vi "BassybassMode.vi"(8 "error in":errorcluster) -> ()   [LabVIEW 2018]
doc: "This VI runs in parallel to other tasks. It can contain as many user-defined periodic loops as you need. These can carry out PID or other sorts of timed response."
uses:
  <vilib>/Platform/TimedLoop/XDataNode/timing_clust.ctl
  <vilib>/Platform/TimedLoop/XDataNode/nitl_modes.ctl
  <vilib>/Platform/TimedLoop/XDataNode/wakeup.ctl
  <vilib>/addons/control/pid/pid.llb/PID (DBL).vi
  <vilib>/platform/TimedLoop/XDataNode/XDataNode.xnode
  <vilib>/addons/control/pid/NI_PID_pid.lvlib
  <vilib>/Platform/TimedLoop/XDataNode/XDNodeRunTimeDep.lvlib
  <vilib>/Rock Robotics/Network Tables/NT Read Numeric Array.vi
panel:
  out "Distance (in)":dbl(slide) scale=14.0..50.0
  in  "XY Tail":i32=10
  out "XY Graph":cluster{dbl[], dbl[]}(graph)
  in  "Moving Avg Size":i32=4
  out "X":cluster{"Numeric":dbl, dbl}(graph)
  out "Z":cluster{"Numeric":dbl, dbl}(graph)
  out "Avg Z":dbl
  out "Avg X":dbl
  out "Cam Tran Array":dbl[](array[numeric])
  out "Yaw Wrap":dbl(graph)=90.04595407731806
  out "Cal Status":T1={"Mag"={"[0]"=FALSE, "[1]"=FALSE, "[2]"=FALSE, "[3]"=TRUE}, "Acc"={"[0]"=TRUE, "[1]"=FALSE, "[2]"=FALSE, "[3]"=FALSE}, "Gyro"={"[0]"=TRUE, "[1]"=FALSE, "[2]"=FALSE, "[3]"=FALSE}, "Sys"={"[0]"=FALSE, "[1]"=FALSE, "[2]"=FALSE, "[3]"=TRUE}, "Status"=TRUE}
  out "Pitch":dbl(graph)=-3.2290155569329033
  out "Roll":dbl(graph)=-0.6325886584475758
  in  "Tab Control":T2(tab)=enum."Sonar"
  out "Sonar Late?":bool
  in  "Period 2":i64=5
  out "Sonar Left":cluster{dbl, dbl}(graph)={10.58349501, 10.58349501}
  in  "PID Sonar":T3={"proportional gain (Kc)"=0.035, "integral time (Ti, min)"=0.0, "derivative time (Td, min)"=0.001} {"derivative time (Td, min)" format="%.5f"; "integral time (Ti, min)" format="%.3f"; "proportional gain (Kc)" format="%.3f"}
  in  "clamp 2":cluster{"output high":dbl, "output low":dbl}={"output high"=0.65, "output low"=-0.65} {"output low" format="%.2f"; "output high" format="%.2f"}
  in  "Standoff (in)":dbl=12.0 format="%.2f"
  out "Sonar error":dbl=1.41650499
  out "Sonar PID":cluster{"setpoint":dbl, "Filtered":dbl, i16}(graph)={"setpoint"=12.0, "Filtered"=10.58349501, 0}
  out "Strobe":bool
  in  "Enc?":bool
  in  "hi limit":dbl=200.0
  out "Mode":bool=TRUE
  out "OOR":bool
  in  "Rate Thresh":dbl=60.0 format="%#_13g"
  out "Arrived 3":bool
  in  "Tol (in) 3":dbl=1.1
  in  "Tol (sec) 3":dbl=0.25 format="%#_13g"
  out "Error 3":dbl=1.41650499
  in  "range 3":cluster{"output high":dbl, "output low":dbl}={"output high"=0.4, "output low"=-0.4} {"output low" format="%.2f"; "output high" format="%.2f"}
  in  "PID IMU 2":T3={"proportional gain (Kc)"=0.035, "integral time (Ti, min)"=0.0, "derivative time (Td, min)"=0.0001} {"derivative time (Td, min)" format="%.5f"; "integral time (Ti, min)" format="%.3f"; "proportional gain (Kc)" format="%.3f"}
  out "Snap Goal":dbl=90.0
  in  "IMU steer?":bool
  in  "w/Joy?":bool=TRUE
  in  "DRIVE?":bool=TRUE
  out "CRD":dbl=-0.007874015748031496
  out "CLD":dbl=-0.007874015748031496
  in  "Negate PID":bool=TRUE
  in  "Hyster":dbl=0.1 format="%#_13g"
  out "Stimulus / Response":cluster{"process variable":dbl, "Yaw":dbl}(graph)={"process variable"=0.0, "Yaw"=0.5729700440447533}
  in  "Read Enable":T4={"Cal Status"=TRUE, "Orientation"=TRUE, "Gyro"=FALSE, "Accelerometer"=FALSE, "Quanterion"=FALSE, "Accel Mode"=enum."Linear", "Magnetometer"=FALSE, "Register Mode"=enum."Quaternion"}
  in  "range 2":cluster{"output high":dbl, "output low":dbl}={"output high"=0.4, "output low"=-0.4} {"output low" format="%.2f"; "output high" format="%.2f"}
  in  "PID IMU":T3={"proportional gain (Kc)"=0.035, "integral time (Ti, min)"=0.0, "derivative time (Td, min)"=0.0001} {"derivative time (Td, min)" format="%.5f"; "integral time (Ti, min)" format="%.3f"; "proportional gain (Kc)" format="%.3f"}
  in  "reset IMU":bool
  out "error":dbl=-0.5729700440447533
  out "Yaw":dbl(graph)=13.384364068810942
  out "Turn CCW":bool=TRUE
  out "Turn CW":bool
  out "Turn":dbl=-0.5729700440447533
  out "Goal":dbl
  # "Larger values move goal\nfurther in direction of travel"
  # "Diagnostics Only"
  # "2016 Bot values:\nP=0.080, I=0.008, D=0.002"
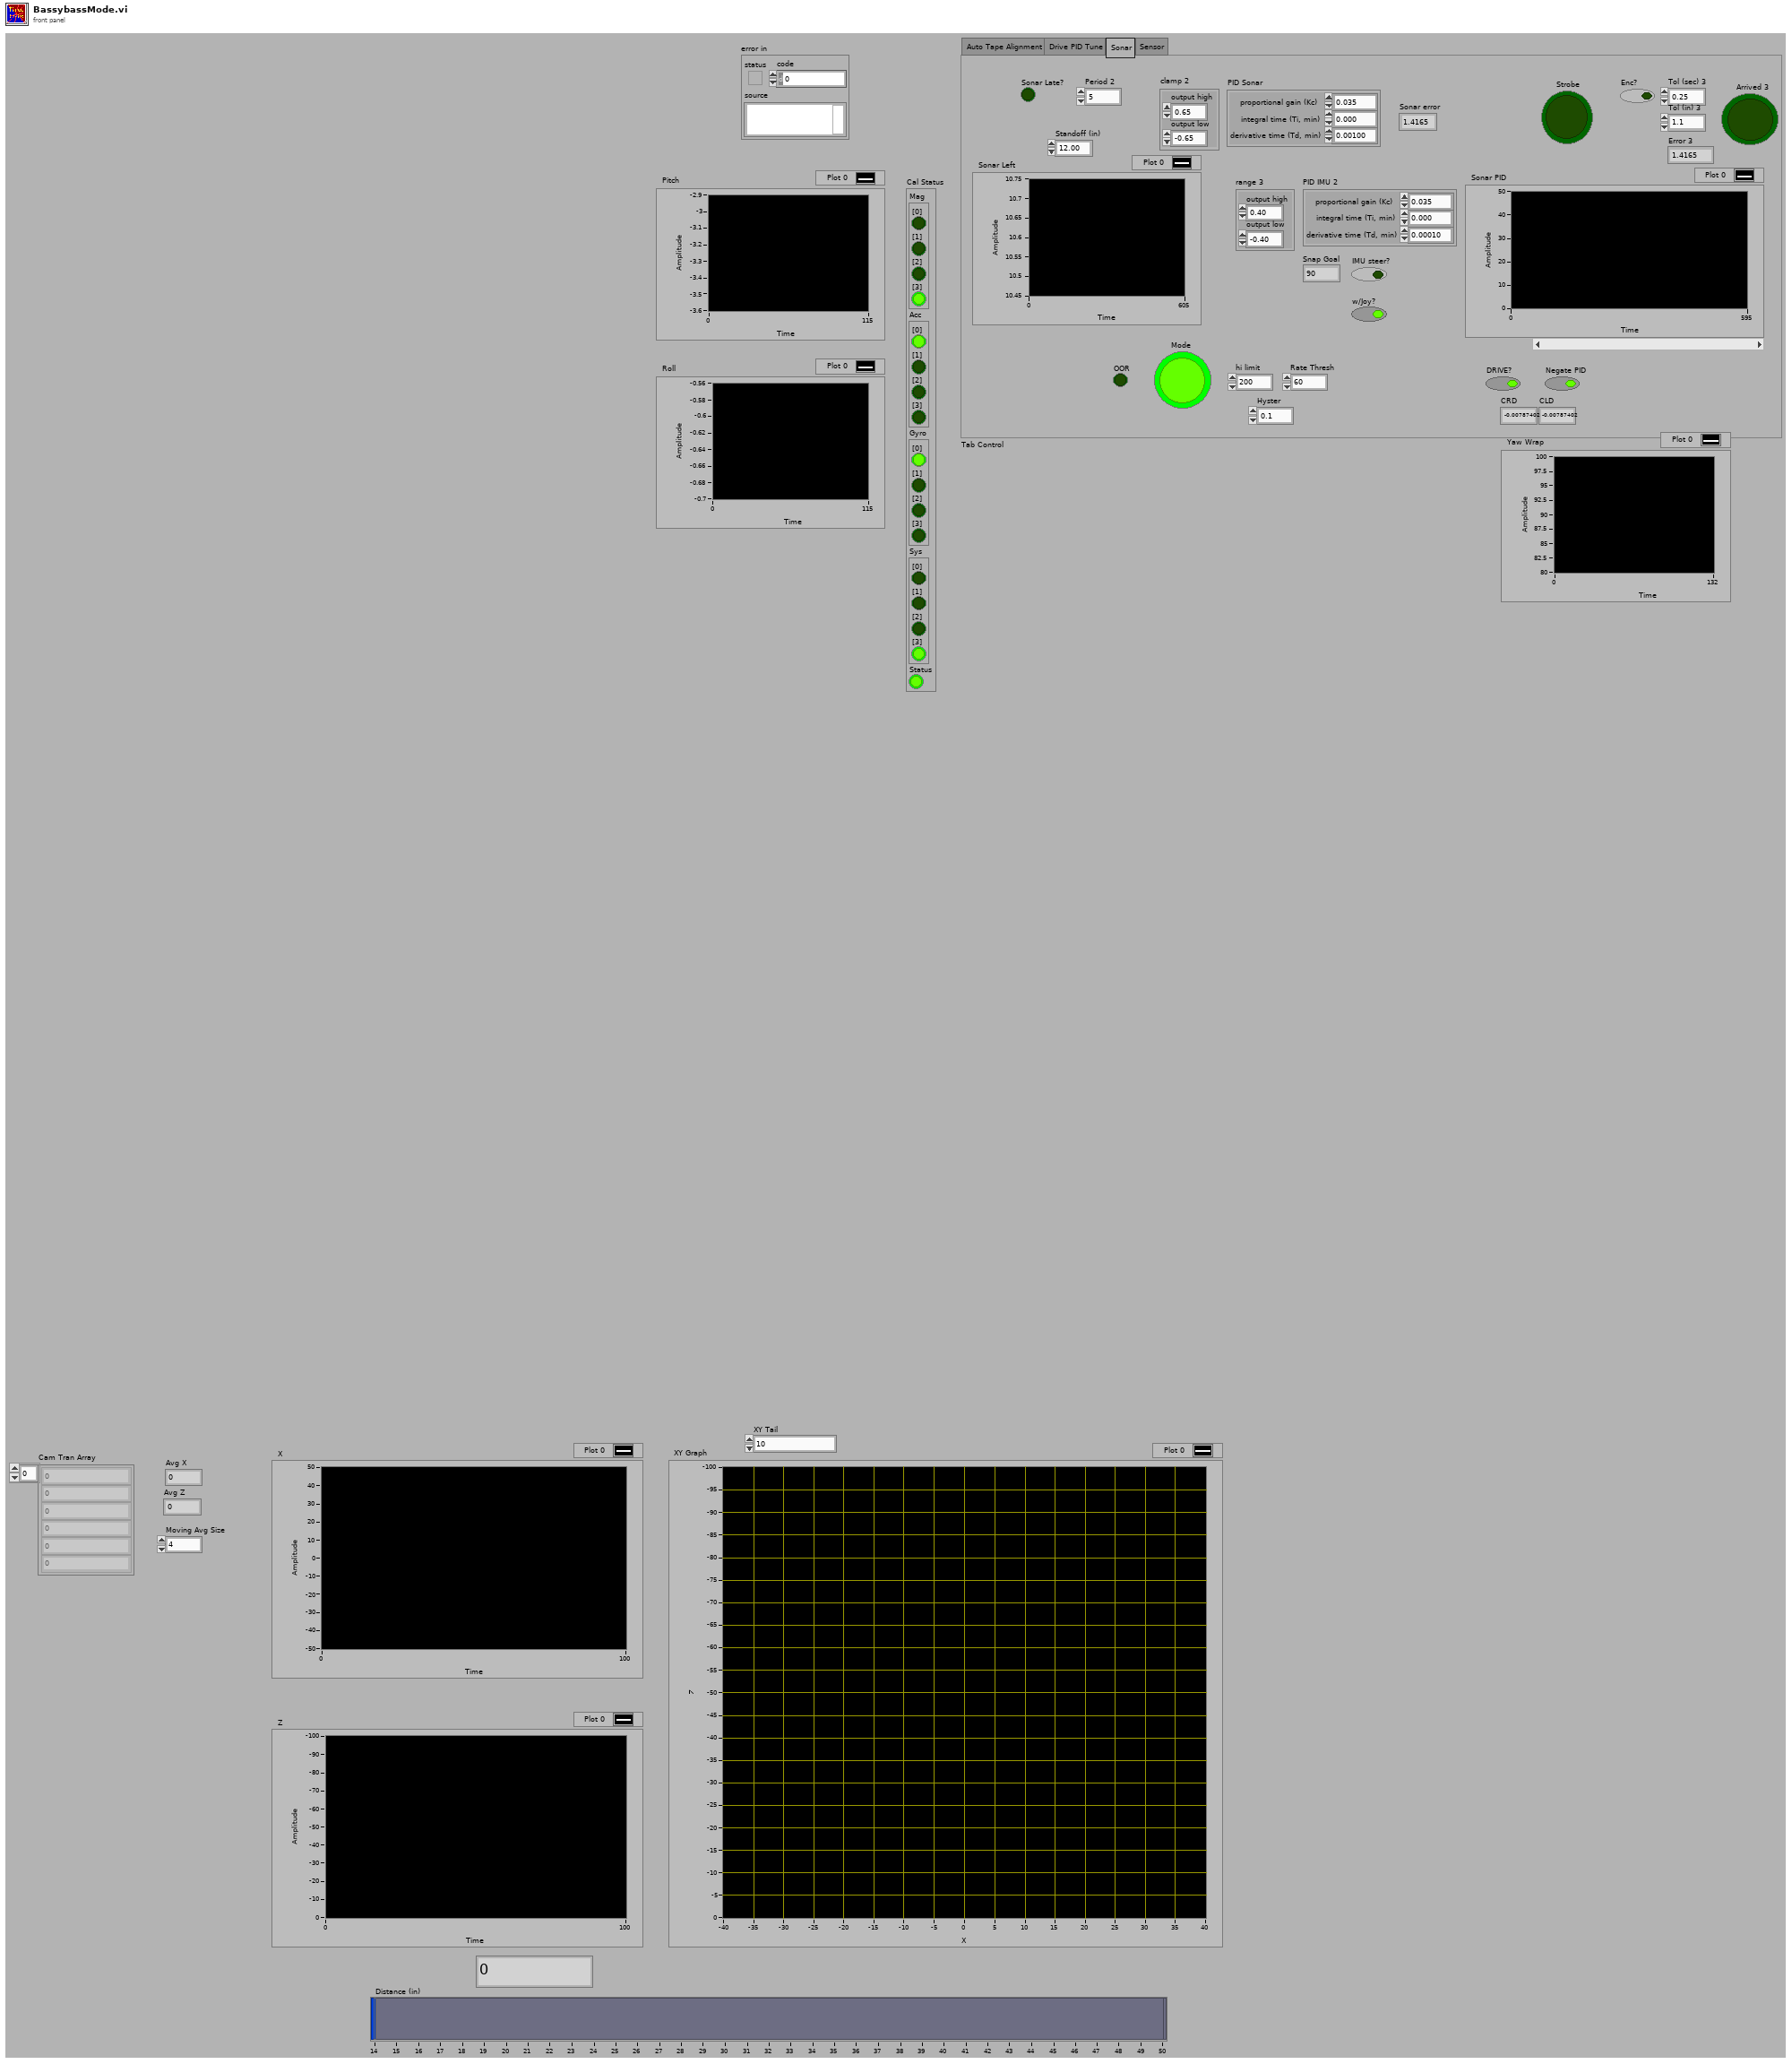
[diagram p1: front panel]
types:
  T1 = cluster{"Mag":cluster{"[0]":bool, "[1]":bool, "[2]":bool, "[3]":bool}, "Acc":cluster{"[0]":bool, "[1]":bool, "[2]":bool, "[3]":bool}, "Gyro":cluster{"[0]":bool, "[1]":bool, "[2]":bool, "[3]":bool}, "Sys":cluster{"[0]":bool, "[1]":bool, "[2]":bool, "[3]":bool}, "Status":bool}
  T2 = enum32{"Auto Tape Alignment", "Drive PID Tune", "Sonar", "Sensor"}
  T3 = cluster{"proportional gain (Kc)":dbl, "integral time (Ti, min)":dbl, "derivative time (Td, min)":dbl}
  T4 = cluster{"Cal Status":bool, "Orientation":bool, "Gyro":bool, "Accelerometer":bool, "Quanterion":bool, "Accel Mode":enum8{"Raw Data", "Linear", "Gravity"}, "Magnetometer":bool, "Register Mode":enum8{"Euler", "Quaternion"}}
  T5 = typedef "XDNodeRunTimeDep.lvlib/timing_clust.ctl" = cluster{"Expected End [f-1]":u64, "Actual End [f-1]":u64, "Finished Late? [f-1]":bool, "Expected End [i-1]":u64, "Actual End [i-1]":u64, "Finished Late? [i-1]":bool, "Expected Start [i]":u64, "Actual Start [i]":u64, "Expected Start [f]":u64, "Actual Start [f]":u64, "Source Name":string, "Structure Name":string, "Period":i64, "Deadline":i64, "Offset":i64, "Start":i64, "Priority":i32, "Timeout":i32, "Mode":T6, "Wakeup Reason":T7, "Error":errorcluster, "Source Type":string, "Secondary Source Type":string, "Global End Time":u64, "Global Start Time":u64, "Frame Duration":u64, "Iteration Duration":u64, "Assigned CPU":i32, "I/O Scan Engine Mode":u32}
  T6 = typedef "XDNodeRunTimeDep.lvlib/nitl_modes.ctl" = enum32{"No Change", "Process missed periods, maintain original phase", "Discard missed periods, maintain original phase", "Process missed periods, ignore original phase", "Discard missed periods, ignore original phase"}
  T7 = typedef "XDNodeRunTimeDep.lvlib/wakeup.ctl" = enum32{"Normal", "Aborted", "Asynchronous wakeup", "Timing source error", "Timed loop error", "Timeout"}
  T8 = typedef "WPI_AnalogChannelDevRef.ctl" = cluster{"DevStatus":errorcluster, "Analog Channel":T9}
  T9 = typedef "FPGA_AIChannel.ctl" = enum8{"AI 0", "AI 1", "AI 2", "AI 3", "AI MXP 0", "AI MXP 1", "AI MXP 2", "AI MXP 3", "Invalid"}
  T10 = typedef "ImuDevRef.ctl" = cluster{"I2CDevRef":T11, "Valid Cal File?":bool}
  T11 = typedef "WPI_I2CDevRef.ctl" = cluster{"DevStatus":errorcluster, "Device Address":u8, "Handle":i32, "I2C Bus":T12}
  T12 = typedef "i2c_bus.ctl" = enum16{"I2C On-Board", "I2C MXP", "Invalid"}
  T13 = cluster{"Yaw":dbl, "Roll":dbl, "Pitch":dbl, "Yaw Wind":dbl, "Roll Wind":dbl, "Pitch Wind":dbl}
  T14 = cluster{"Standoff (in)":dbl, "Filtered":dbl, i16}
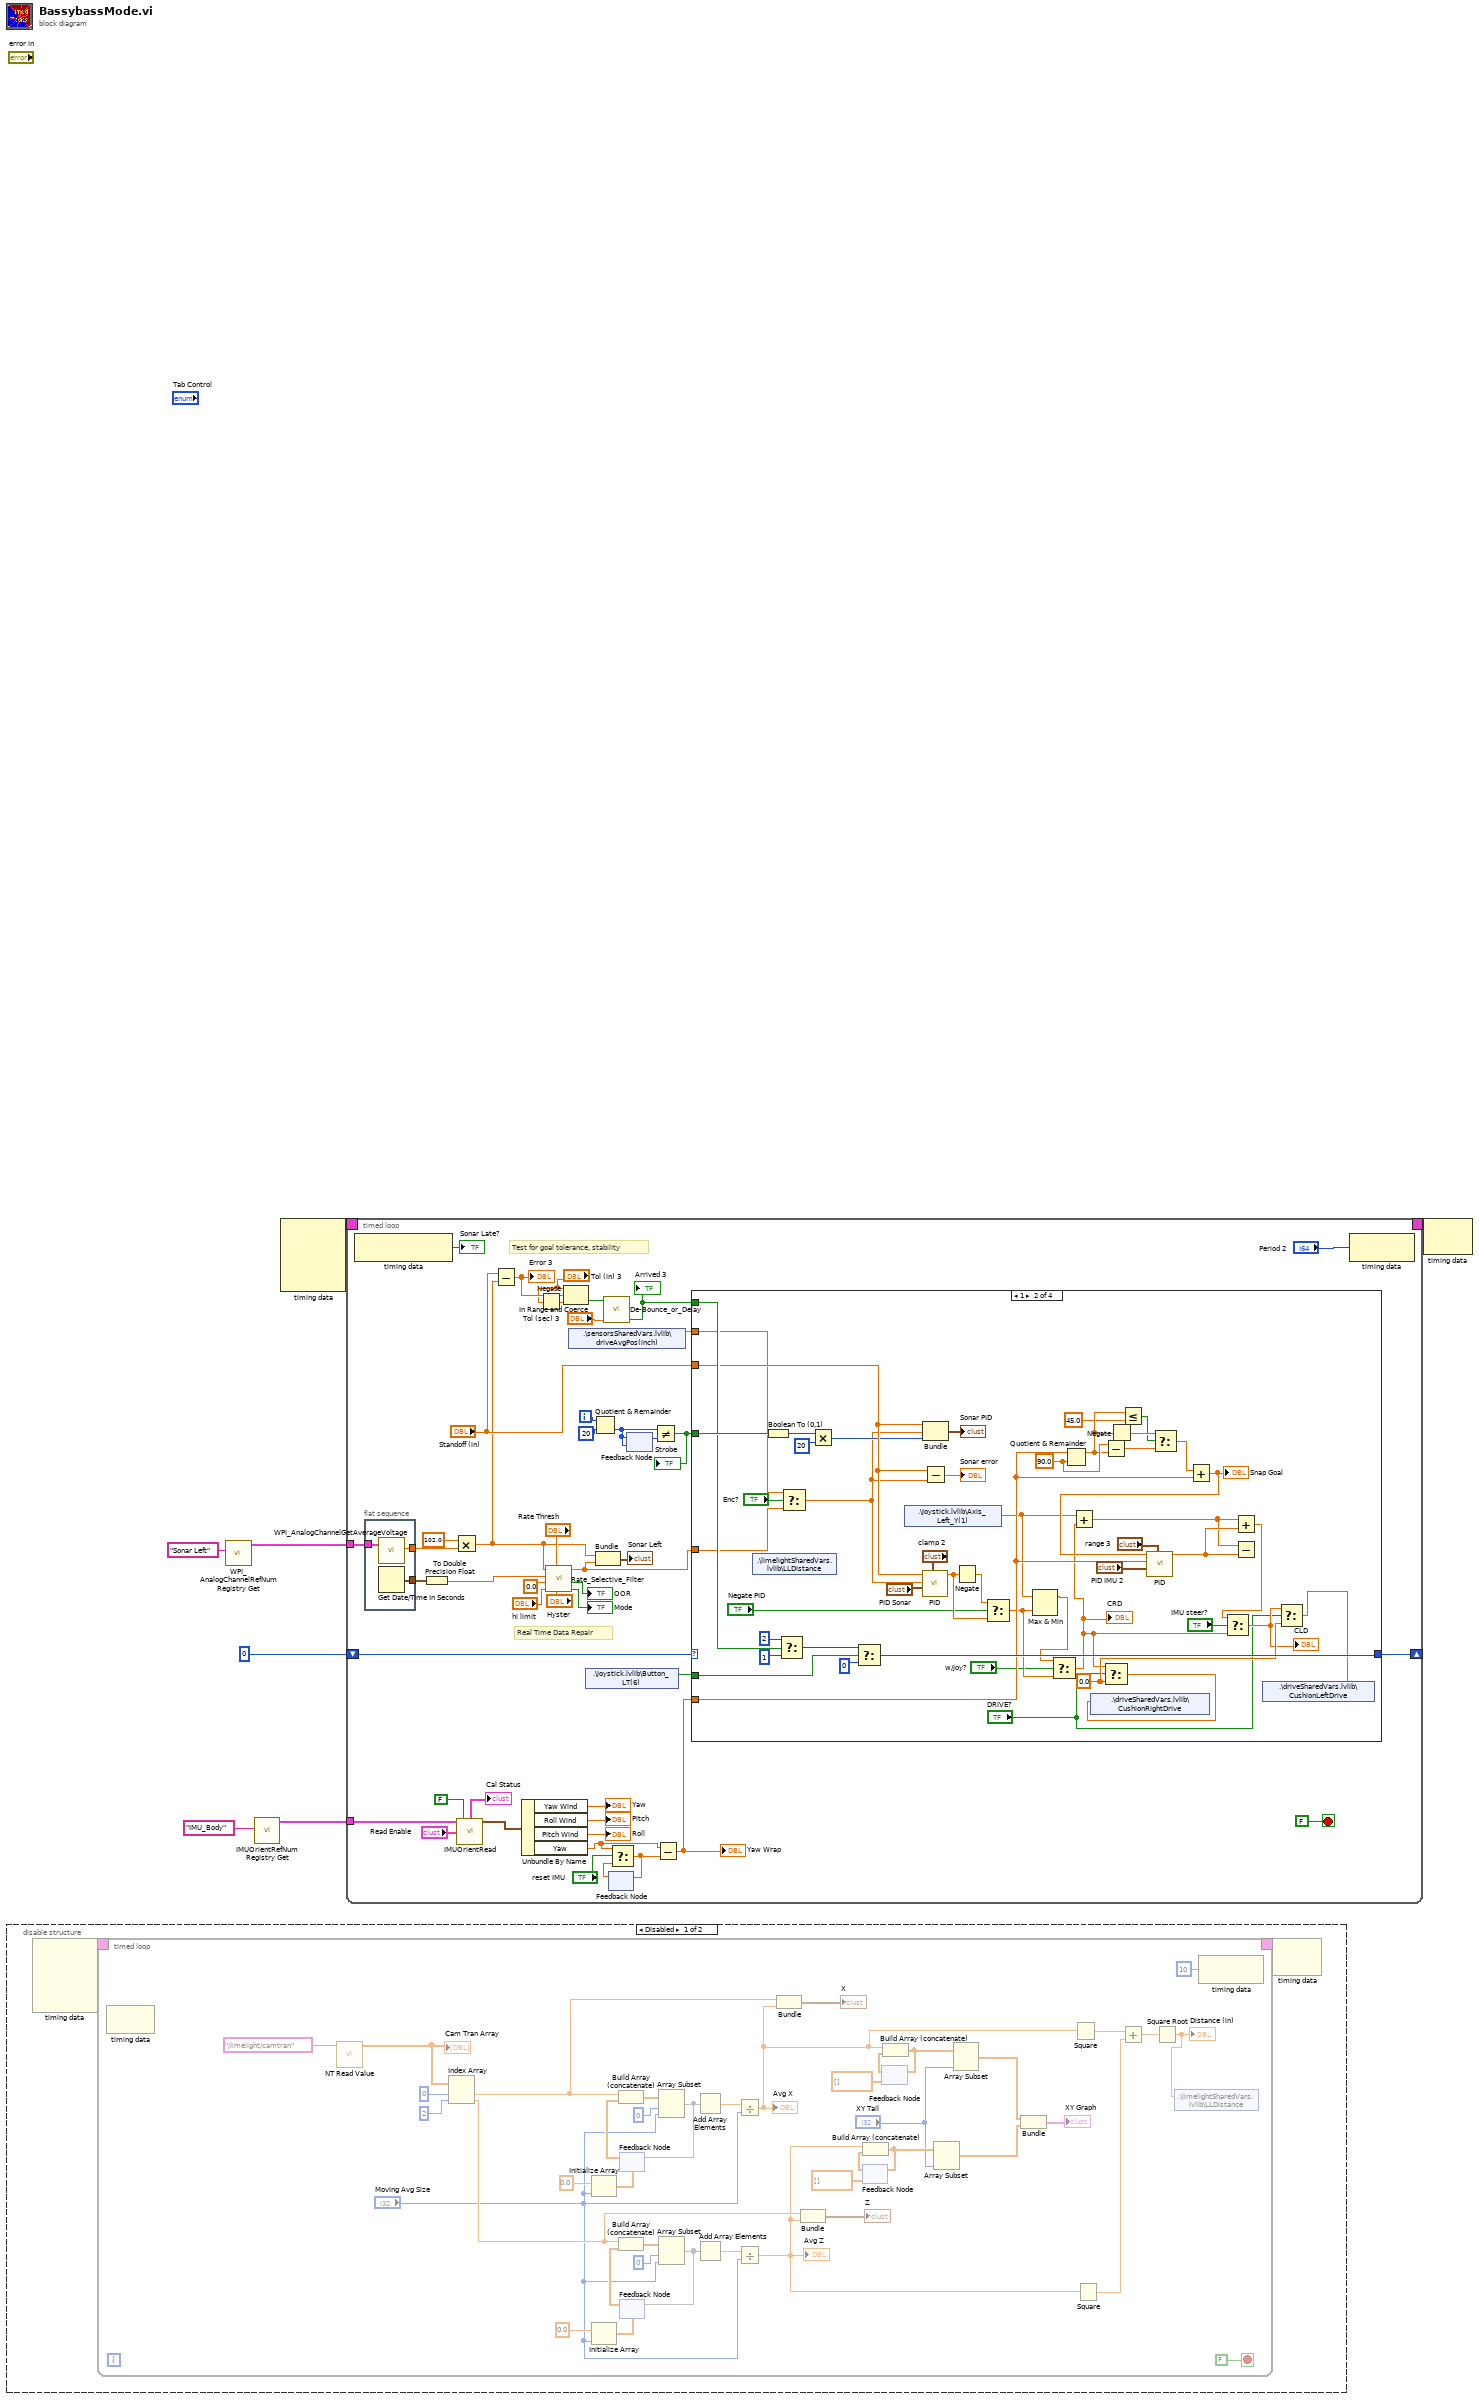
[diagram p0: block diagram]
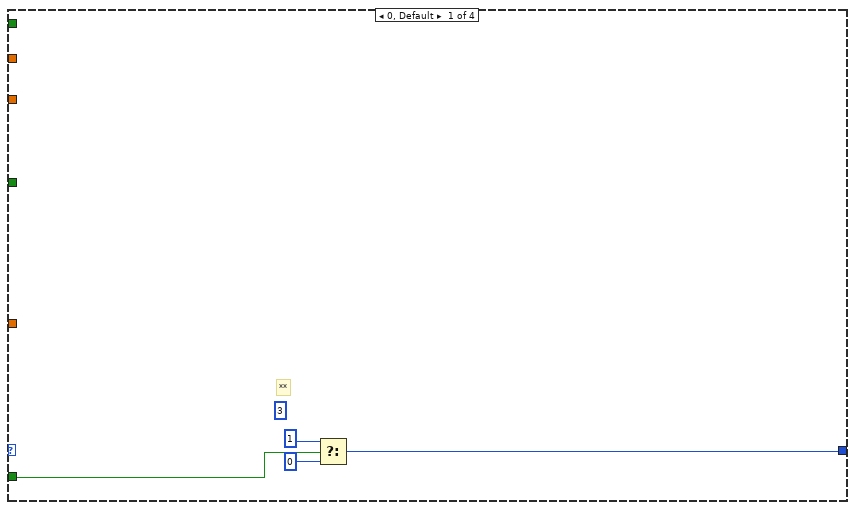
[diagram p3: hidden frame]
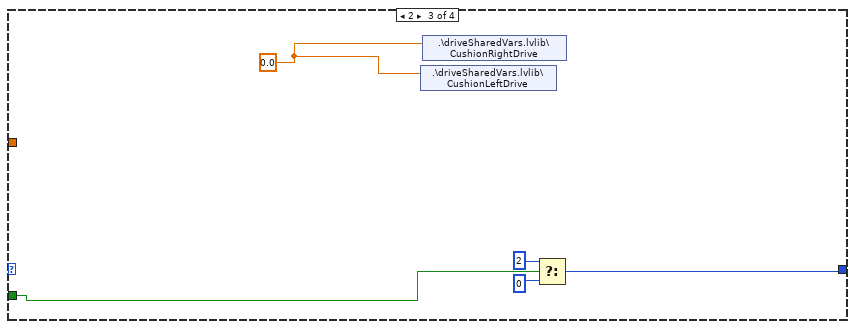
[diagram p4: hidden frame]
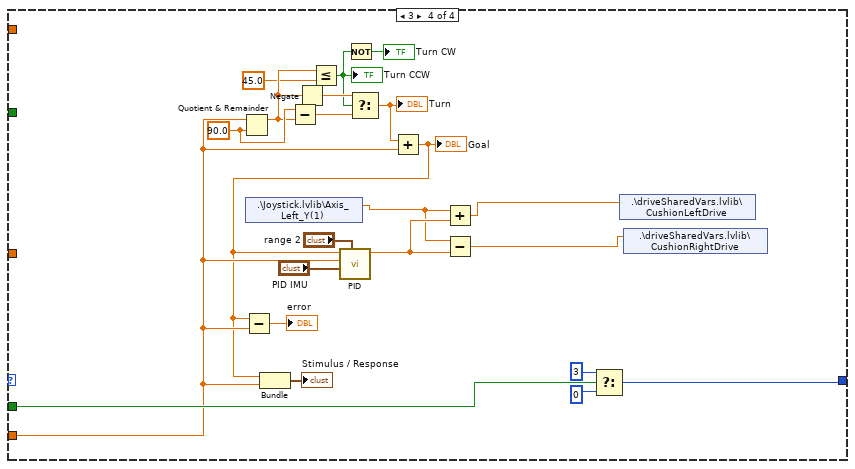
[diagram p5: hidden frame]
diagram:
  n1 = disable-structure shown="Disabled" {
    frame Disabled {
      n2 = node-c288() -> (w9:T5)  [unwired: 4 in]
      n3 = timed-loop {
        timing: w9 -> [_]
        timing-out: [_] -> w8
        stop <- FALSE stop-if-true
        n4 = node-c288() -> ()  [unwired: 1 in, 1 out]
        n5 = call-poly <vilib>:"NT Read Value.vi"("Name"="/limelight/camtran") -> ("Numeric Array"=w49:dbl[])  [unwired: 9 in, 1 out]
        "Cam Tran Array" <- w49
        n6 = Index Array(array=w49, index #1=0 ("index"), index #2=2 ("index")) -> (element #1=w42:dbl, element #2=w30:dbl)
        n7 = Initialize Array(0.0 ("element"), "Moving Avg Size") -> (w45:dbl[])
        n8 = Initialize Array(0.0 ("element"), "Moving Avg Size") -> (w36:dbl[])
        n9 = feedback #1(w45) -> (w46:dbl[])
        n10 = Build Array (concatenate)(w42, w46) -> (w40:dbl[])
        n11 = feedback #2(w36) -> (w37:dbl[])
        n12 = Build Array (concatenate)(w30, w37) -> (w33:dbl[])
        n13 = Array Subset(array=w40, index=0, length="Moving Avg Size") -> (w38:dbl[])
        n14 = feedback-in #1(w38) -> ()
        n15 = Array Subset(array=w33, index=0, length="Moving Avg Size") -> (w31:dbl[])
        n16 = feedback-in #2(w31) -> ()
        n17 = Add Array Elements(numeric array=w38) -> (sum=w43:dbl)
        n18 = Add Array Elements(numeric array=w31) -> (sum=w34:dbl)
        n19 = Divide(x=w43, y="Moving Avg Size") -> (x/y=w17:dbl)
        "Avg X" <- w17
        n20 = Divide(x=w34, y="Moving Avg Size") -> (x/y=w16:dbl)
        "Avg Z" <- w16
        n21 = Bundle("Numeric"=w42, w17) -> (→"X":cluster{"Numeric":dbl, dbl})  [unwired: 1 in]
        n22 = Bundle("Numeric"=w30, w16) -> (→"Z":cluster{"Numeric":dbl, dbl})  [unwired: 1 in]
        n23 = feedback #3(dbl[] []) -> (w27:dbl[])
        n24 = Build Array (concatenate)(w16, w27) -> (w26:dbl[])
        n25 = feedback-in #3(w26) -> ()
        n26 = feedback #4(dbl[] []) -> (w24:dbl[])
        n27 = Build Array (concatenate)(w17, w24) -> (w23:dbl[])
        n28 = feedback-in #4(w23) -> ()
        n29 = Array Subset(array=w26, length="XY Tail") -> (w20:dbl[])  [unwired: 1 in]
        n30 = Array Subset(array=w23, length="XY Tail") -> (w19:dbl[])  [unwired: 1 in]
        n31 = Bundle(w19, w20) -> (→"XY Graph":cluster{dbl[], dbl[]})  [unwired: 1 in]
        n32 = Square(x=w17) -> (x^2=w15:dbl)
        n33 = Square(x=w16) -> (x^2=w14:dbl)
        n34 = Add(x=w15, y=w14) -> (x+y=w13:dbl)
        n35 = Square Root(x=w13) -> (sqrt(x)=w11:dbl)
        "Distance (in)" <- w11
        n36 = shared-variable ".\\limelightSharedVars.lvlib\\LLDistance"(w11) -> ()  [unwired: 1 in, 1 out]
        n37 = node-c288(i64 10 ("Period")) -> ()  [unwired: 1 out]
      }
      n38 = node-c288(w8) -> ()  [unwired: 1 out]
    }
    frame Enabled {
    }
  }
  n39 = call <vilib>:"WPI_AnalogChannelRefNum Registry Get.vi"("refnum name"="Sonar Left") -> ("AIDeviceRef"=w4:T8)  [unwired: 9 in, 1 out]
  n40 = call <userlib>:"IMUOrientRefNum Registry Get.vi"("refnum name"="IMU_Body") -> ("IMUDevRef out"=w1:T10)  [unwired: 9 in, 1 out]
  n41 = node-c288() -> (w7:T5)  [unwired: 4 in]
  n42 = timed-loop {
    timing: w7 -> [_]
    timing-out: [_] -> w6
    tunnel: w4 -> [w100]
    shift-right: [w98] -> _
    shift-left: 0 -> [w97]
    tunnel: w1 -> [w74]
    i -> [w92]
    stop <- FALSE stop-if-true
    # "Real Time Data Repair"
    # "Test for goal tolerance, stability"
    n43 = node-c288() -> (→"Sonar Late?":bool)  [unwired: 1 in]
    n44 = flat-sequence {
      tunnel: [w105] -> w83
      tunnel: w100 -> [w104]
      tunnel: [w103] -> w89
      frame #0 {
        n45 = call <vilib>:"WPI_AnalogChannelGetAverageVoltage.vi"("AIDeviceRef"=w104) -> ("Voltage"=w105:dbl)  [unwired: 8 in, 2 out]
        n46 = Get Date/Time In Seconds() -> (seconds since 1Jan1904=w103:timestamp)
      }
    }
    n47 = To Double Precision Float(number=w89) -> (double precision float=w88:dbl)
    n48 = Multiply(x=102.0, y=w83) -> (x*y=w70:dbl)
    n49 = call <userlib>:"IMUOrientRead.vi"("IMU Dev Ref"=w74, "Orient Reset (Wind)"=FALSE, "Read Enable"="Read Enable") -> ("Cal Status"=→"Cal Status":T1, "Orient Y/R/P"=w63:T13)  [unwired: 5 in, 6 out]
    n50 = Subtract(x="Standoff (in)", y=w70) -> (x-y=w82:dbl)
    "Error 3" <- w82
    n51 = Unbundle By Name(w63) -> ("Yaw Wind"=→"Yaw":dbl, "Roll Wind"=→"Pitch":dbl, "Pitch Wind"=→"Roll":dbl, "Yaw"=w57:dbl)
    n52 = Negate(x="Tol (in) 3") -> (-x=w81:dbl)
    n53 = call <userlib>:"Rate_Selective_Filter.vi"("Hyster"="Hyster", "Rate Thresh"="Rate Thresh", "hi limit"="hi limit", "lo limit"=0.0, "Time"=w88, "Distance"=w70) -> ("Mode"=→"Mode":bool, "OOR"=→"OOR":bool, "Filtered"=w68:dbl)  [unwired: 1 in]
    n54 = In Range and Coerce(upper limit="Tol (in) 3", x=w82, lower limit=w81) -> (In Range?=w79:bool)  [unwired: 1 out]
    n55 = shared-variable ".\\sensorsSharedVars.lvlib\\driveAvgPos(inch)"() -> (w71:dbl)  [unwired: 1 in, 1 out]
    n56 = shared-variable ".\\Joystick.lvlib\\Button_LT(6)"() -> (w96:bool)  [unwired: 1 in, 1 out]
    n57 = Quotient & Remainder(x=w92, y=20) -> (floor(x/y)=w95:i32)  [unwired: 1 out]
    n58 = Bundle(w70, "Filtered"=w68) -> (→"Sonar Left":cluster{dbl, "Filtered":dbl})  [unwired: 1 in]
    n59 = call <userlib>:"De-Bounce_or_Delay.vi"("Eval Period (sec)"="Tol (sec) 3", "Signal Input"=w79) -> ("Stable"=w77:bool)  [unwired: 9 in]
    "Arrived 3" <- w77
    n60 = feedback #5() -> (w61:dbl)  [unwired: 1 in]
    n61 = Select(t=w57, s="reset IMU", f=w61) -> (s? t:f=w60:dbl)
    n62 = feedback-in #5(w60) -> ()
    n63 = feedback #6(w95) -> (w94:i32)
    n64 = feedback-in #6(w95) -> ()
    n65 = Not Equal?(x=w95, y=w94) -> (x != y?=w76:bool)
    "Strobe" <- w76
    n66 = Subtract(x=w57, y=w60) -> (x-y=w73:dbl)
    "Yaw Wrap" <- w73
    n67 = case shown="1" w97 {
      tunnel: [w108 w155 w160 w181] -> w98
      tunnel: w96 -> [w106 w154 w159 w182]
      tunnel: "Standoff (in)" -> [_ w141 _ _]
      tunnel: w71 -> [_ w137 _ _]
      tunnel: w76 -> [_ w149 _ _]
      tunnel: w68 -> [_ w110 _ _]
      tunnel: w77 -> [_ w145 _ _]
      tunnel: w73 -> [_ w125 _ w168]
      frame 0, Default {
        (unwired) 3
        # "**"
        n68 = Select(t=1, s=w106, f=0) -> (s? t:f=w108:i32)
      }
      frame 1 {
        w116 = 0.0 ("f")
        w131 = 90.0 ("y")
        n69 = shared-variable ".\\limelightSharedVars.lvlib\\LLDistance"() -> ()  [unwired: 1 in, 2 out]
        n70 = Boolean To (0,1)(Boolean=w149) -> (0, 1=w150:i16)
        n71 = Select(t=2, s=w145, f=1) -> (s? t:f=w142:i32)
        n72 = Select(t=w137, s="Enc?", f=w110) -> (s? t:f=w138:dbl)
        n73 = Multiply(x=w150, y=i16 20) -> (x*y=w139:i16)
        n74 = Select(t=w142, s=w154, f=0) -> (s? t:f=w155:i32)
        n75 = shared-variable ".\\Joystick.lvlib\\Axis_Left_Y(1)"() -> (w118:dbl)  [unwired: 1 in, 1 out]
        n76 = call-poly <vilib>:"PID.vi"("output range"="clamp 2", "PID gains"="PID Sonar", "process variable"=w138, "setpoint"=w141) -> ("output"=w153:dbl)  [unwired: 6 in, 1 out]
        n77 = Bundle("Standoff (in)"=w141, "Filtered"=w138, w139) -> (→"Sonar PID":T14)  [unwired: 1 in]
        n78 = Subtract(x=w141, y=w138) -> (x-y=→"Sonar error":dbl)
        n79 = Negate(x=w153) -> (-x=w152:dbl)
        n80 = Select(t=w152, s="Negate PID", f=w153) -> (s? t:f=w121:dbl)
        n81 = Max & Min(x=w118, y=w121) -> (max(x,y)=w122:dbl)  [unwired: 1 out]
        n82 = Select(t=w122, s="w/Joy?", f=w121) -> (s? t:f=w113:dbl)
        "CRD" <- w113
        n83 = Quotient & Remainder(x=w125, y=w131) -> (x-y*floor(x/y)=w130:dbl)  [unwired: 1 out]
        n84 = Add(x=w118, y=w113) -> (x+y=w119:dbl)
        n85 = Subtract(x=w131, y=w130) -> (x-y=w129:dbl)
        n86 = Select(t=w113, s="DRIVE?", f=w116) -> (s? t:f=w115:dbl)
        n87 = shared-variable ".\\driveSharedVars.lvlib\\CushionRightDrive"(w115) -> ()  [unwired: 1 in, 1 out]
        n88 = Negate(x=w130) -> (-x=w133:dbl)
        n89 = Less Or Equal?(x=w130, y=45.0) -> (x <= y?=w126:bool)
        n90 = Select(t=w133, s=w126, f=w129) -> (s? t:f=w132:dbl)
        n91 = Add(x=w132, y=w125) -> (x+y=w127:dbl)
        "Snap Goal" <- w127
        n92 = call-poly <vilib>:"PID.vi"("output range"="range 3", "PID gains"="PID IMU 2", "process variable"=w125, "setpoint"=w127) -> ("output"=w134:dbl)  [unwired: 6 in, 1 out]
        n93 = Add(x=w119, y=w134) -> (x+y=w124:dbl)
        n94 = Select(t=w124, s="IMU steer?", f=w113) -> (s? t:f=w114:dbl)
        "CLD" <- w114
        n95 = Subtract(x=w119, y=w134) -> ()  [unwired: 1 out]
        n96 = Select(t=w114, s="DRIVE?", f=w116) -> (s? t:f=w117:dbl)
        n97 = shared-variable ".\\driveSharedVars.lvlib\\CushionLeftDrive"(w117) -> ()  [unwired: 1 in, 1 out]
      }
      frame 2 {
        w158 = 0.0 ("Left Drive")
        n98 = shared-variable ".\\driveSharedVars.lvlib\\CushionLeftDrive"(w158) -> ()  [unwired: 1 in, 1 out]
        n99 = shared-variable ".\\driveSharedVars.lvlib\\CushionRightDrive"(w158) -> ()  [unwired: 1 in, 1 out]
        n100 = Select(t=2, s=w159, f=0) -> (s? t:f=w160:i32)
      }
      frame 3 {
        w173 = 90.0 ("y")
        n101 = Quotient & Remainder(x=w168, y=w173) -> (x-y*floor(x/y)=w172:dbl)  [unwired: 1 out]
        n102 = shared-variable ".\\Joystick.lvlib\\Axis_Left_Y(1)"() -> (w163:dbl)  [unwired: 1 in, 1 out]
        n103 = Subtract(x=w173, y=w172) -> (x-y=w171:dbl)
        n104 = Negate(x=w172) -> (-x=w175:dbl)
        n105 = Less Or Equal?(x=w172, y=45.0) -> (x <= y?=w166:bool)
        "Turn CCW" <- w166
        n106 = Not(x=w166) -> (.not. x?=→"Turn CW":bool)
        n107 = Select(t=w175, s=w166, f=w171) -> (s? t:f=w174:dbl)
        "Turn" <- w174
        n108 = Add(x=w174, y=w168) -> (x+y=w167:dbl)
        "Goal" <- w167
        n109 = Subtract(x=w167, y=w168) -> (x-y=→"error":dbl)
        n110 = Bundle(w167, w168) -> (→"Stimulus / Response":cluster{dbl, dbl})  [unwired: 1 in]
        n111 = call-poly <vilib>:"PID.vi"("output range"="range 2", "PID gains"="PID IMU", "process variable"=w168, "setpoint"=w167) -> ("output"=w176:dbl)  [unwired: 6 in, 1 out]
        n112 = Add(x=w163, y=w176) -> (x+y=w165:dbl)
        n113 = Subtract(x=w163, y=w176) -> (x-y=w164:dbl)
        n114 = Select(t=3, s=w182, f=0) -> (s? t:f=w181:i32)
        n115 = shared-variable ".\\driveSharedVars.lvlib\\CushionLeftDrive"(w165) -> ()  [unwired: 1 in, 1 out]
        n116 = shared-variable ".\\driveSharedVars.lvlib\\CushionRightDrive"(w164) -> ()  [unwired: 1 in, 1 out]
      }
    }
    n117 = node-c288("Period 2") -> ()  [unwired: 1 out]
  }
  n118 = node-c288(w6) -> ()  [unwired: 1 out]
